vi "test Deployment NI-SWITCH and RaF CD.vi"(8 "error in (no error)":errorcluster, 11 "TestCase in":refnum<class "NI-SWITCH System Tests.lvclass">) -> (0 "error out":errorcluster, 3 "TestCase out":refnum<class "NI-SWITCH System Tests.lvclass">)   [LabVIEW 2017, in "NI-SWITCH System Tests.lvclass"]
uses:
  NI-SWITCH System Tests.lvclass
  C:/Users/nitest/Desktop/Git 2017/niveristand-custom-device-testing-tools/VeriStandTestCase/VeriStandTestCase.lvclass
  06447cec-b57b-42f3-8866-b6c62ecd6767.vi
  <vilib>/NI Veristand/Execution/Workspace/NI VeriStand - Get Multiple Channel Values.vi
  <vilib>/addons/_JKI Toolkits/VI Tester/TestCase.llb/TestCase.lvclass
  <vilib>/NI VeriStand/Execution/Workspace/NI_VS Workspace ExecutionAPI.lvlib
  C:/Program Files (x86)/National Instruments/LabVIEW 2017/vi.lib/addons/_JKI Toolkits/VI Tester/TestCase.llb/TestCase.lvclass
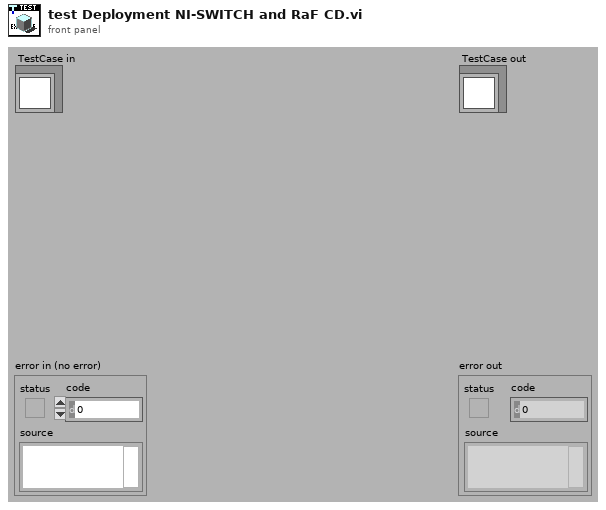
[diagram p1: front panel]
types:
  T1 = typedef "NI_VS Workspace ExecutionAPI.lvlib/WorkspaceAPI.ctl" = refnum<k24>
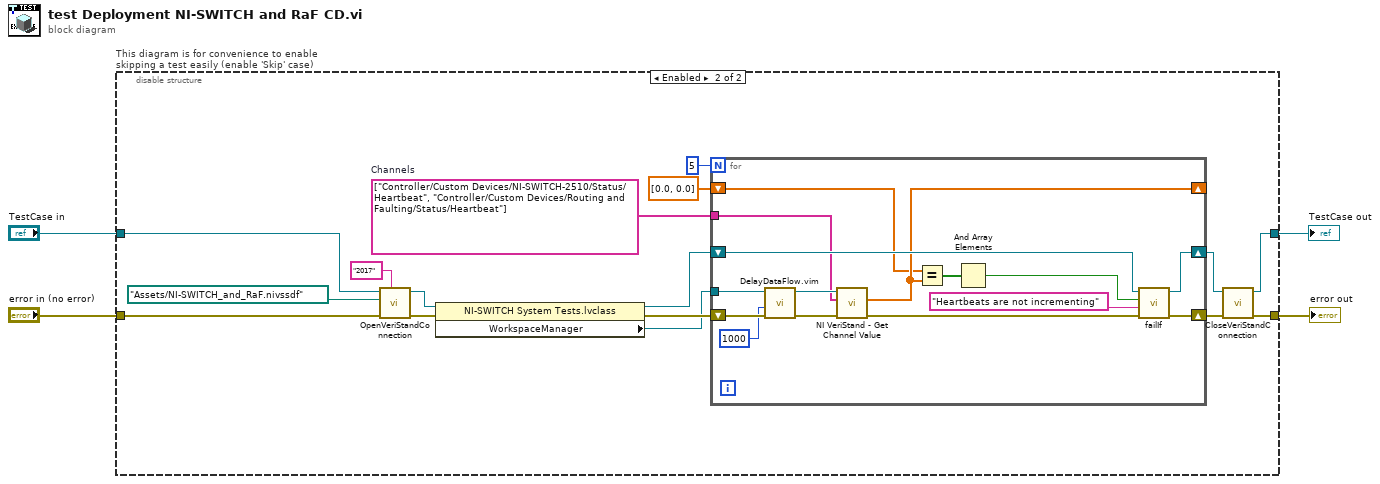
[diagram p0: block diagram]
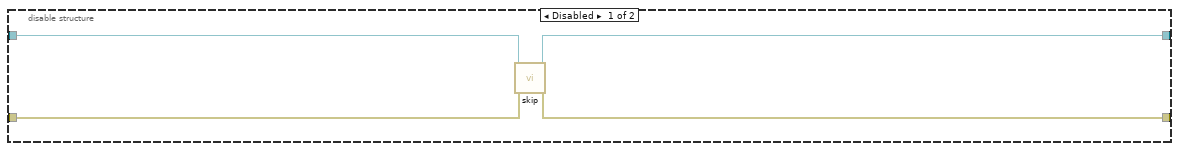
[diagram p2: hidden frame]
diagram:
  n1 = disable-structure "This diagram is for convenience to enable skipping a test easily (enable 'Skip' case)" shown="Enabled" {
    disable-tunnel: "TestCase in" -> [w8 w24]
    disable-tunnel: [w7 w22] -> w1
    disable-tunnel: [w6 w21] -> w3
    disable-tunnel: "error in (no error)" -> [w5 w23]
    frame Disabled {
      n2 = call <vilib>:"skip.vi"("error in (no error)"=w5, "TestCase in"=w8) -> ("error out"=w6:errorcluster, "TestCase out"=w7:refnum<class "NI-SWITCH System Tests.lvclass">)  [unwired: 8 in]
    }
    frame Enabled {
      w11 = string[] ["Controller/Custom Devices/NI-SWITCH-2510/Status/Heartbeat", "Controller/Custom Devices/Routing and Faulting/Status/Heartbeat"]  # Channels
      n3 = call-dynamic "OpenVeriStandConnection.vi"("Minimum VeriStand Version (2016)"="2017" ("Minimum VeriStand Version (2015)"), "error in (no error)"=w23, "System Definition File"=path "Assets/NI-SWITCH_and_RaF.nivssdf", "VeriStand Test Case in"=w24) -> ("error out"=w17:errorcluster, "VeriStand Test Case out"=w18:refnum<class "NI-SWITCH System Tests.lvclass">)  [unwired: 5 in, 1 out]
      n4 = property class="NI-SWITCH System Tests.lvclass"(reference=w18, error in=w17) -> (reference out=w13:refnum<class "NI-SWITCH System Tests.lvclass">, error out=w16:errorcluster, "WorkspaceManager"=w14:T1)
      n5 = for {
        N: 5 -> [_]
        shift-right: [w33] -> w15
        shift-left: w16 -> [w29]
        tunnel: w14 -> [w38]
        shift-right: [w31] -> w12
        shift-left: w13 -> [w32]
        tunnel: w11 -> [w30]
        shift-right: [w26] -> _
        shift-left: dbl[] [0.0, 0.0] ("Values") -> [w25]
        n6 = call "DelayDataFlow.vim"("value in"=w29, "milliseconds to wait"=u32 1000) -> ("value out"=w28:errorcluster)  [unwired: 2 in, 1 out]
        n7 = call-poly <vilib>:"NI VeriStand - Get Channel Value.vi"("error in (no error)"=w28, "Channels"=w30, "WorkspaceManager in"=w38) -> ("error out"=w34:errorcluster, "Values"=w26:dbl[])  [unwired: 6 in, 1 out]
        n8 = Equal?(x=w25, y=w26) -> (x = y?=w37:bool[])
        n9 = And Array Elements(Boolean array=w37) -> (logical AND=w36:bool)
        n10 = call-dynamic "failIf.vi"("error in (no error)"=w34, "message (\"\")"="Heartbeats are not incrementing" ("message (\"\")"), "fail"=w36, "TestCase in"=w32) -> ("error out"=w33:errorcluster, "TestCase out"=w31:refnum<class "NI-SWITCH System Tests.lvclass">)  [unwired: 6 in]
      }
      n11 = call-dynamic "CloseVeriStandConnection.vi"("error in (no error)"=w15, "VeriStand Test Case in"=w12) -> ("error out"=w21:errorcluster, "VeriStand Test Case out"=w22:refnum<class "NI-SWITCH System Tests.lvclass">)  [unwired: 8 in]
    }
  }
  "error out" <- w3
  "TestCase out" <- w1
